vi "GetParameterDefaults.vi"(8 "error in (no error)":errorcluster, 11 "CGrapherDGML in":refnum<class "CGrapherDGML.lvclass">) -> (0 "error out":errorcluster, 1 "Parameter defaults":string, 3 "CGrapherDGML out":refnum<class "CGrapherDGML.lvclass">)   [LabVIEW 2020, in "DefaultExtensions.lvlib" / "CGrapherDGML.lvclass"]
uses:
  CGrapherDGML.lvclass
  Private/Parameters.ctl
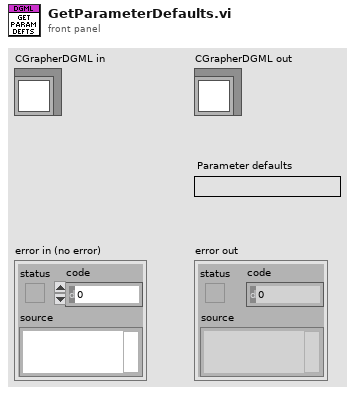
[diagram p1: front panel]
types:
  T1 = typedef "DefaultExtensions.lvlib/CGrapherDGML.lvclass/Parameters.ctl" = cluster{"Path":string, "Expand containers":bool, "Group by folder":bool, "Show full paths":bool, "Source folder?":bool, "Target folder?":bool, "Add virtual folders?":bool}
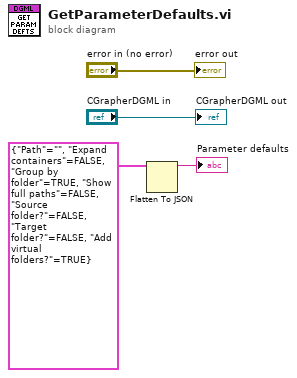
[diagram p0: block diagram]
diagram:
  n1 = Flatten To JSON(anything=T1 {"Path"="", "Expand containers"=FALSE, "Group by folder"=TRUE, "Show full paths"=FALSE, "Source folder?"=FALSE, "Target folder?"=FALSE, "Add virtual folders?"=TRUE} ("Parameters")) -> (JSON string=→"Parameter defaults":string)  [unwired: 2 in, 1 out]
  "error out" <- "error in (no error)"
  "CGrapherDGML out" <- "CGrapherDGML in"
